vi "Destroy.vi"(0 "reference in":refnum<class "DqmhModuleDiagramGraph.lvclass">, 5 "error in (no error)":errorcluster) -> (19 "error out":errorcluster)   [LabVIEW 2020, in "DqmhModuleDiagramGraph.lvclass"]
doc: "Destroys a ClassDiagramGraph object created with a ClassDiagramGraph constructor VI.\n\n[GOOP 2.1]"
uses:
  <resource>/Framework/Providers/Open_GDS/UML/DqmhModuleDiagramGraph_class/DqmhModuleDiagramGraph.lvclass
  <resource>/Framework/Providers/Open_GDS/UML/Graph_class/Graph.lvclass
panel:
  out "reference out":refnum<class "DqmhModuleDiagramGraph.lvclass">
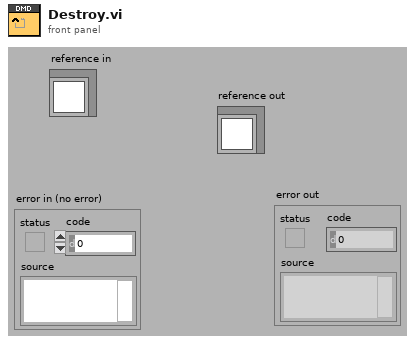
[diagram p1: front panel]
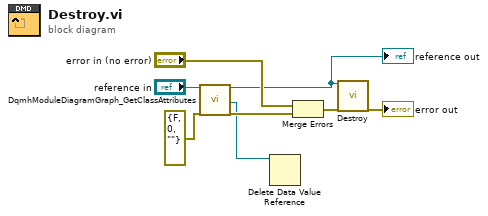
[diagram p0: block diagram]
diagram:
  n1 = call <resource>:"DqmhModuleDiagramGraph_GetClassAttributes.vi"("reference in"="reference in", "error in (no error)"=errorcluster {"status"=FALSE, "code"=0, "source"=""}) -> ("reference out"=w3:refnum<class "DqmhModuleDiagramGraph.lvclass">, "Class attribute Reference"=w1:refnum<data-value>, "error out"=w4:errorcluster)  [unwired: 15 out]
  "reference out" <- w3
  n2 = Delete Data Value Reference(data value reference=w1) -> ()  [unwired: 1 in, 2 out]
  n3 = Merge Errors("error in (no error)", w4) -> (w2:errorcluster)
  n4 = call-parent "Destroy.vi"("reference"=w3, "error in (no error)"=w2) -> ("error out"=→"error out":errorcluster)  [unwired: 17 in]
